vi "Do.vi"(8 "error in":errorcluster, 10 "Actor in":refnum<class "Actor.lvclass">, 11 "Send New Chirp MSG":refnum<class "Send New Chirp MSG.lvclass">) -> (0 "error out":errorcluster, 2 "Actor out":refnum<class "Actor.lvclass">)   [LabVIEW 2015, in "ePAS Library.lvlib" / "Send New Chirp MSG.lvclass"]
doc: "(<B>Filename</B>: Actor Framework.lvlib:Message.lvclass:Do.vi)\n\nDefines what a message does when it is received by an actor. Generally, a message instructs an actor to invoke one of its methods. By default, this method does nothing. A child class must override it to define behavior. Create a child class by using the Actor Framework Message Maker dialog box."
uses:
  Send New Chirp MSG.lvclass
  Instr Actor.lvclass
  PAS/Commands/Load New Speaker Chirp/Load New Speaker Chirp.lvclass
  reusable/Command/Command.lvclass
  SuperActor/SuperActor.lvclass
  reusable/Session APIs/CVT/CVT.lvclass
  <vilib>/ActorFramework/Actor/Actor.lvclass
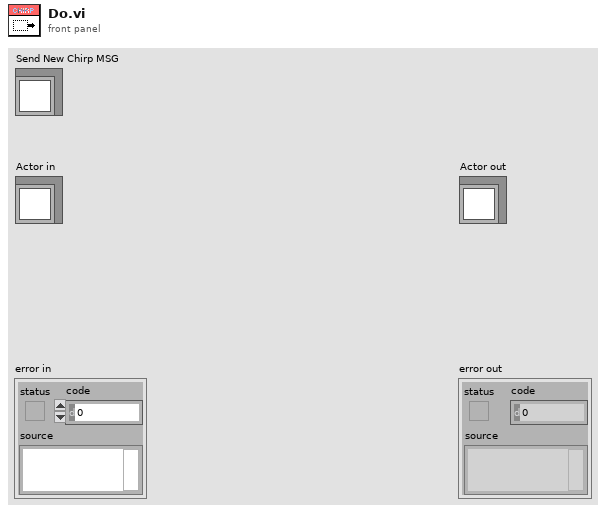
[diagram p1: front panel]
types:
  T1 = typedef "Session - Root.lvclass/Session Handle.ctl" = refnum<data-value>
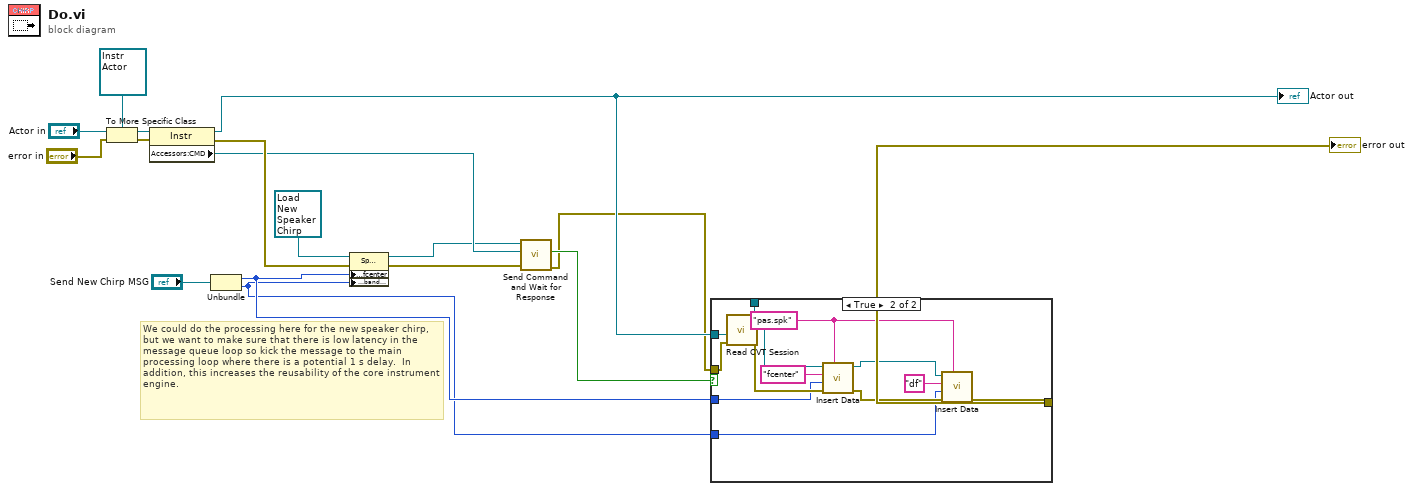
[diagram p0: block diagram]
diagram:
  # "We could do the processing here for the new speaker chirp, but we want to make sure that there is low latency in the message queue loop so kick the message to the main processing loop where there is a potential 1 s delay.  In addition, this increases the reusability of the core instrument engine."
  n1 = To More Specific Class(target class=refnum<class "Instr Actor.lvclass"> refnum ("Instrument Lib:Instr"), reference="Actor in", error in="error in") -> (specific class reference=w14:refnum<class "Instr Actor.lvclass">, error out=w12:errorcluster)
  n2 = property class="Instr"(reference=w14, error in=w12) -> (reference out=w5:refnum<class "Instr Actor.lvclass">, error out=w10:errorcluster, "Accessors:CMD"=w9:refnum<queue>)
  "Actor out" <- w5
  n3 = Unbundle("Send New Chirp MSG") -> (w4:i16, w1:i16)
  n4 = property class="Speaker Chirp"(reference=refnum<class "Load New Speaker Chirp.lvclass"> refnum ("Speaker Chirp"), error in=w10, "Accessors:fcenter"=w4, "Accessors:bandwidth"=w1) -> (reference out=w8:refnum<class "Load New Speaker Chirp.lvclass">, error out=w7:errorcluster)
  n5 = call "Send Command and Wait for Response.vi"("error in"=w7, "cmd queue"=w9, "CMD in"=w8) -> ("error out"=w3:errorcluster, "cmd good?"=w6:bool)  [unwired: 6 in, 1 out]
  n6 = case shown="True" w6 {
    tunnel: w5 -> [w19 w32]
    tunnel: [w19 w30] -> _
    tunnel: w3 -> [w18 w29]
    tunnel: [w18 w20] -> w2
    tunnel: w4 -> [_ w26]
    tunnel: w1 -> [_ w21]
    frame False {
    }
    frame True {
      w24 = "pas.spk" ("Group")
      n7 = call "Read CVT Session.vi"("error in (no error)"=w29, "Ex Nested in"=w32) -> ("error out"=w28:errorcluster, "Session Handle"=w31:T1, "Ex Nested out"=w30:refnum<class "Instr Actor.lvclass">)  [unwired: 7 in]
      n8 = call "Insert Data.vi"("Group"=w24, "error in"=w28, "Data"=w26, "tag"="fcenter", "CVT Session In"=w31) -> ("error out"=w25:errorcluster, "CVT Session Out"=w23:T1)  [unwired: 5 in]
      n9 = call "Insert Data.vi"("Group"=w24, "error in"=w25, "Data"=w21, "tag"="df", "CVT Session In"=w23) -> ("error out"=w20:errorcluster)  [unwired: 5 in, 1 out]
    }
  }
  "error out" <- w2
